vi "mathscriptreceiver.vi"(11 "Array in":cdb[](array[numeric])) -> (3 "Array out":cdb[](array[numeric]))   [LabVIEW 2013]
uses:
  <vilib>/imath/engines/lvmath2/RunTimeEngine/ErrorHandling/NIMS_Finalize Error.vi
  <vilib>/imath/engines/lvmath2/RunTimeEngine/Managers/WorkSpace/UID Generator.vi
  <vilib>/imath/engines/lvmath2/RunTimeEngine/Managers/SymbolTable/Clear UID.vi
  <vilib>/imath/engines/lvmath2/RunTimeEngine/NodeEndStatement/NIMS_NodeEndStatement_Output.vi
  <instcachedir>/0/NIMS_NodeEndStatement_Output_53EC0D466D134D7ABD903AC30B43404B.lvgen/NIMS_NodeEndStatement_Output_53EC0D466D134D7ABD903AC30B43404B_005.vi
  <vilib>/imath/engines/lvmath2/RunTimeEngine/RangeToken/NIMS_Range.vi
  <instcachedir>/0/NIMS_Range_7481B155BEE341ECA0F59DDB444E2C09.lvgen/NIMS_Range_7481B155BEE341ECA0F59DDB444E2C09_000.vi
  <vilib>/imathl/engines/lvmath/Functions/Error Handling/Create Error.vi
  <vilib>/imath/engines/lvmath2/RunTimeEngine/IndexRead/NIMS V(R2).vi
  <instcachedir>/0/NIMS V(R2)_C76619605A0E4E9F8B2FA9389712AC47.lvgen/NIMS V(R2)_C76619605A0E4E9F8B2FA9389712AC47_000.vi
  <vilib>/imath/engines/lvmath2/RunTimeEngine/BuiltInFunctions/mirrorh/NIMS_mirrorh(GRowV).vi
  <instcachedir>/0/NIMS_mirrorh(GRowV)_B6A8CC4EAFBA4F9A82A59460D67BDFF0.lvgen/NIMS_mirrorh(GRowV)_B6A8CC4EAFBA4F9A82A59460D67BDFF0_000.vi
  <vilib>/imath/engines/lvmath2/RunTimeEngine/RunTimeType/NIMS_RunTimeType_From StrictType (excl LVString).vi
  <instcachedir>/0/NIMS_RunTimeType_From StrictType (excl LVString)_4DEE718D6EB74582AA20236969C084FC.lvgen/NIMS_RunTimeType_From StrictType (excl LVString)_4DEE718D6EB74582AA20236969C084FC_000.vi
  <vilib>/imath/engines/lvmath2/RunTimeEngine/LocalVariableDefStatement/MC_LocalVariableDefStatement_Display.vi
  <vilib>/imath/engines/lvmath2/RunTimeEngine/ErrorHandling/NIMS_Create Error From Enums.vi
  <instcachedir>/0/NIMS_NodeEndStatement_Output_53EC0D466D134D7ABD903AC30B43404B.lvgen/NIMS_NodeEndStatement_Output_53EC0D466D134D7ABD903AC30B43404B_000.vi
  <vilib>/imath/engines/lvmath2/RunTimeEngine/ArithmeticOperatorToken/NIMS_ArithmeticOperator_times.vi
  <instcachedir>/0/NIMS_ArithmeticOperator_times_F6527734CE75451889337B8CE94765C6.lvgen/NIMS_ArithmeticOperator_times_F6527734CE75451889337B8CE94765C6_000.vi
  <vilib>/imath/engines/lvmath2/RunTimeEngine/ArithmeticOperatorToken/NIMS_ArithmeticOperator_plus.vi
  <instcachedir>/0/NIMS_ArithmeticOperator_plus_8A46DAFC24D445C9B2C97B626139369E.lvgen/NIMS_ArithmeticOperator_plus_8A46DAFC24D445C9B2C97B626139369E_004.vi
  <vilib>/imath/engines/lvmath2/RunTimeEngine/ArithmeticOperatorToken/NIMS_ArithmeticOperator_rightdiv.vi
  <instcachedir>/0/NIMS_ArithmeticOperator_rightdiv_C75411BD8BC84A93B6F1C8DA359A92EC.lvgen/NIMS_ArithmeticOperator_rightdiv_C75411BD8BC84A93B6F1C8DA359A92EC_000.vi
  <vilib>/imath/engines/lvmath2/RunTimeEngine/BuiltInFunctions/conv/NIMS_conv(V,V).vi
  <instcachedir>/0/NIMS_conv(V,V)_D3E194F2B5174935BB2368CEB7AAC5A9.lvgen/NIMS_conv(V,V)_D3E194F2B5174935BB2368CEB7AAC5A9_000.vi
  <vilib>/imath/engines/lvmath2/RunTimeEngine/ErrorHandling/NIMS_Error From Error Code.vi
  <vilib>/imath/engines/lvmath2/RunTimeEngine/BuiltInFunctions/numelements/NIMS_numelements.vi
  <instcachedir>/0/NIMS_numelements_A776DA77F73142F68C2F209B523114C5.lvgen/NIMS_numelements_A776DA77F73142F68C2F209B523114C5_004.vi
  <vilib>/imath/engines/lvmath2/RunTimeEngine/BuiltInFunctions/zeros/NIMS_V=zeros(I32,I32).vi
  <vilib>/imath/engines/lvmath2/RunTimeEngine/RangeToken/NIMS_Range_R2 - Float.vi
  <instcachedir>/0/NIMS_Range_R2 - Float_E19924E36A3948A4B33043226480F83C.lvgen/NIMS_Range_R2 - Float_E19924E36A3948A4B33043226480F83C_000.vi
  <vilib>/imath/engines/lvmath2/RunTimeEngine/CommandStatement/MC_CommandStatement_break.vi
  <vilib>/imath/engines/lvmath2/RunTimeSupport/NIMS_Error if Not Equal.vi
  <instcachedir>/0/NIMS_Error if Not Equal_902F5D2649E64F5087A1EF57C55C58AB.lvgen/NIMS_Error if Not Equal_902F5D2649E64F5087A1EF57C55C58AB_000.vi
  <vilib>/imath/engines/lvmath2/RunTimeEngine/IndexRead/NIMS V(S).vi
  <instcachedir>/0/NIMS V(S)_0488751826AF41519A22953C041130DC.lvgen/NIMS V(S)_0488751826AF41519A22953C041130DC_000.vi
  <vilib>/imath/engines/lvmath2/RunTimeEngine/IndexReplace/NIMS V(S)=S.vi
  <instcachedir>/0/NIMS V(S)=S_66A18068148B4981A312229A93EA5C06.lvgen/NIMS V(S)=S_66A18068148B4981A312229A93EA5C06_000.vi
  <vilib>/imath/engines/lvmath2/RunTimeEngine/BuiltInFunctions/round/NIMS_round(DBL-S).vi
  <vilib>/imath/engines/lvmath2/RunTimeEngine/Managers/SymbolTable/NIMS_WorkSpace.lvlib
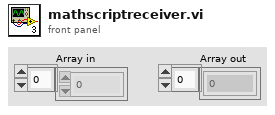
[diagram p1: front panel]
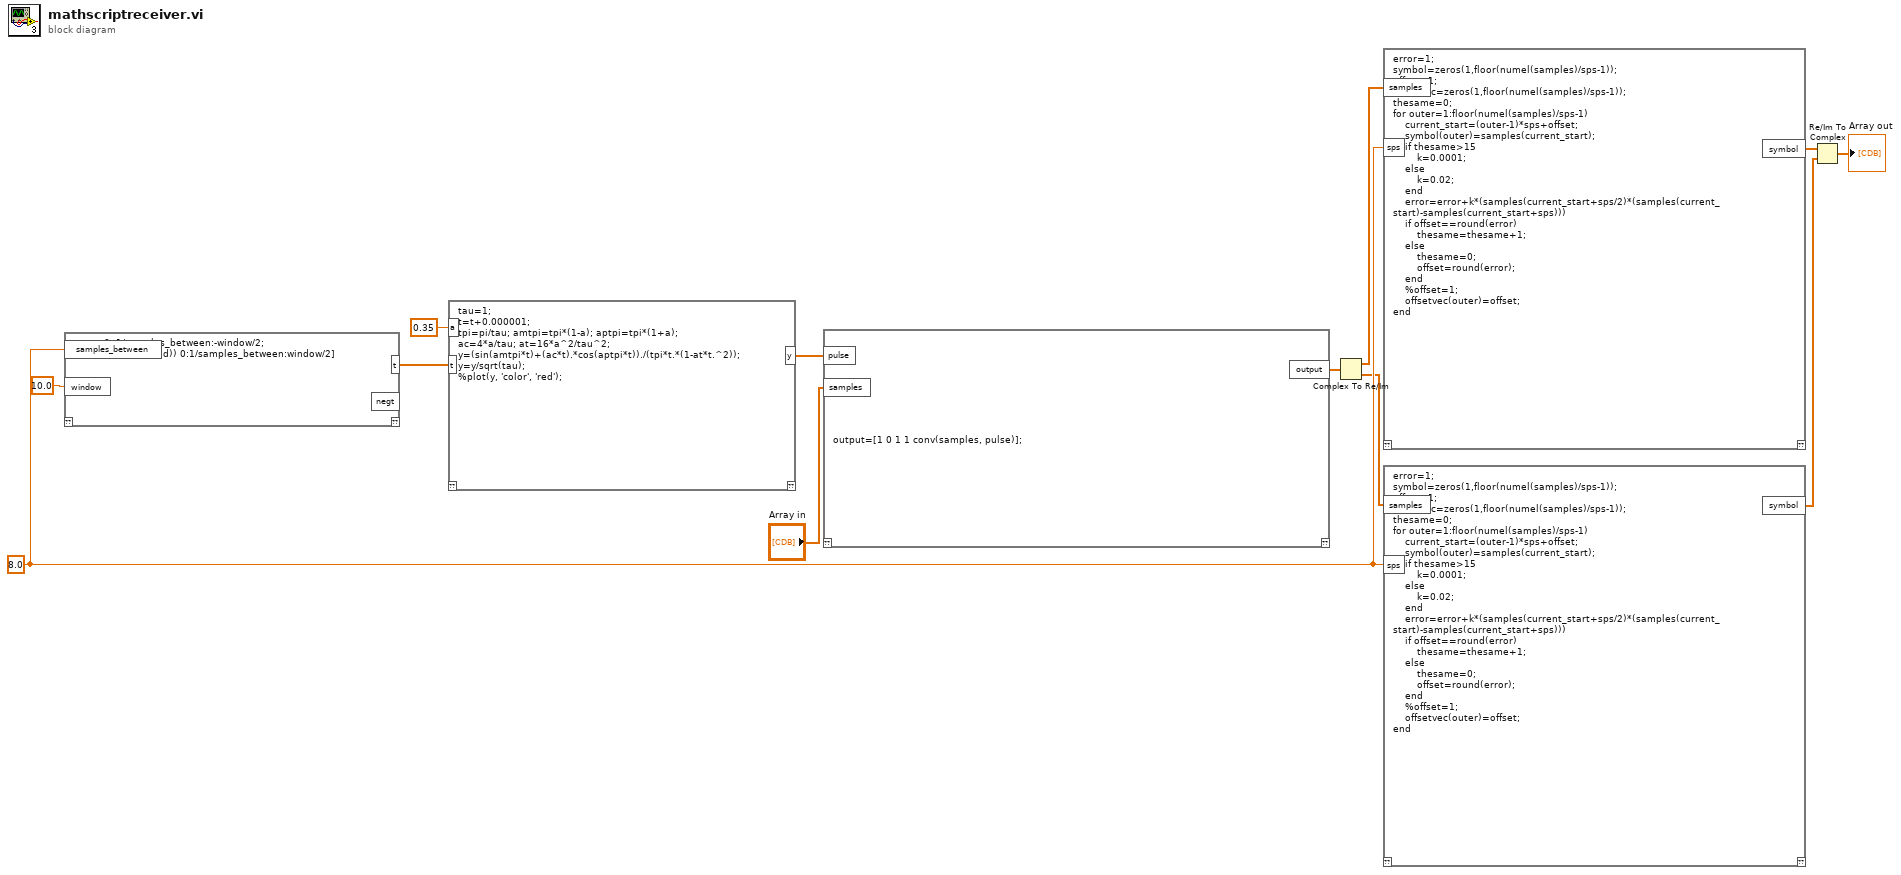
[diagram p0: block diagram]
diagram:
  w8 = 8.0 ("samples_between")
  n1 = mathscript code="negt=0:-1/samples_between:-window/2;\nt=[fliplr(negt(2:end)) 0:1/samples_between:window/2]"("samples_between"=w8, "window"=10.0) -> ("t"=w2:dbl[])  [unwired: 1 in, 2 out]
  n2 = mathscript code="tau=1;\nt=t+0.000001;\ntpi=pi/tau; amtpi=tpi*(1-a); aptpi=tpi*(1+a);\nac=4*a/tau; at=16*a^2/tau^2;\ny=(sin(amtpi*t)+(ac*t).*cos(aptpi*t))./(tpi*t.*(1-at*t.^2));\ny=y/sqrt(tau);\n%plot(y, 'color', 'red');"("a"=0.35, "t"=w2) -> ("y"=w4:cdb[])  [unwired: 1 in, 1 out]
  n3 = mathscript code="output=[1 0 1 1 conv(samples, pulse)];"("pulse"=w4, "samples"="Array in") -> ("output"=w5:cdb[])  [unwired: 1 in, 1 out]
  n4 = Complex To Re/Im(x + iy=w5) -> (x=w6:dbl[], y=w7:dbl[])
  n5 = mathscript code="error=1;\nsymbol=zeros(1,floor(numel(samples)/sps-1));\noffset=1;\noffsetvec=zeros(1,floor(numel(samples)/sps-1));\nthesame=0;\nfor outer=1:floor(numel(samples)/sps-1)\n    current_start=(outer-1)*sps+offset;\n    symbol(outer)=samples(current_start);\n    if thesame>15\n        k=0.0001;\n    else\n        k=0.02;\n    end\n    error=error+k*(samples(current_start+sps/2)*(samples(current_start)-samples(current_start+sps)))\n    if offset==round(error)\n        thesame=thesame+1;\n    else\n        thesame=0;\n        offset=round(error);\n    end\n    %offset=1;\n    offsetvec(outer)=offset;\nend"("samples"=w6, "sps"=w8) -> ("symbol"=w9:dbl[])  [unwired: 1 in, 1 out]
  n6 = mathscript code="error=1;\nsymbol=zeros(1,floor(numel(samples)/sps-1));\noffset=1;\noffsetvec=zeros(1,floor(numel(samples)/sps-1));\nthesame=0;\nfor outer=1:floor(numel(samples)/sps-1)\n    current_start=(outer-1)*sps+offset;\n    symbol(outer)=samples(current_start);\n    if thesame>15\n        k=0.0001;\n    else\n        k=0.02;\n    end\n    error=error+k*(samples(current_start+sps/2)*(samples(current_start)-samples(current_start+sps)))\n    if offset==round(error)\n        thesame=thesame+1;\n    else\n        thesame=0;\n        offset=round(error);\n    end\n    %offset=1;\n    offsetvec(outer)=offset;\nend"("samples"=w7, "sps"=w8) -> ("symbol"=w10:dbl[])  [unwired: 1 in, 1 out]
  n7 = Re/Im To Complex(1:w10, 2:w9) -> (0:→"Array out":cdb[])
